vi "imageToIntensityArray.vi"(2 "errorIn":errorcluster, 3 "image":T1) -> (0 "erorOut":errorcluster, 1 "imageArray":u16[][](array[numeric]))   [LabVIEW 2021]
uses:
  <vilib>/vision/Image Controls.llb/IMAQ Image.ctl
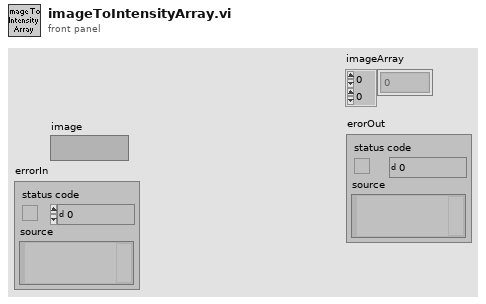
[diagram p1: front panel]
types:
  T1 = typedef "IMAQ Image.ctl" = refnum<image>
  T2 = typedef "Image Type" = u32
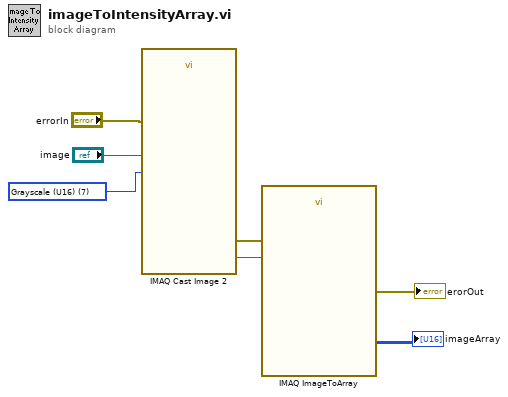
[diagram p0: block diagram]
diagram:
  w5 = T2 7 items=["Grayscale (U8)", "Grayscale (I16)", "Grayscale (SGL)", "Complex (CSG)", "RGB (U32)", "HSL (U32)", "RGB (U64)", "Grayscale (U16)"] ("Image Type")
  n1 = call "IMAQ Cast Image 2"("Image Src"="image", "Image Type"=w5, "error in (no error)"="errorIn") -> ("Image Dst Out"=w7:T1, "error out"=w3:errorcluster)  [unwired: 11 in]
  n2 = call "IMAQ ImageToArray"("error in (no error)"=w3, "Image"=w7) -> ("Image Pixels (U16)"=→"imageArray":u16[][], "error out"=→"erorOut":errorcluster)  [unwired: 2 in, 3 out]
